vi "automatic_step_first_name.vi"(7 "transition_queue":refnum<queue>, 8 "error in (no error)":errorcluster, 10 "data":variant, 11 "recipe_data":variant) -> (0 "error out":errorcluster)   [LabVIEW 2015, in "example_02.lvlib"]
uses:
  example_02.lvlib
  <userlib>/antonio-alexander/lv-recipe-machine/public/_controls/transition.ctl
  _controls/customer.ctl
  <userlib>/antonio-alexander/lv-recipe-machine/lv-recipe-machine.lvlib
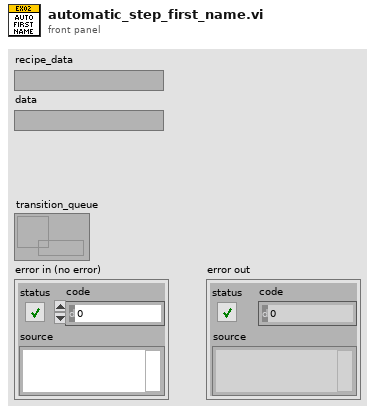
[diagram p1: front panel]
types:
  T1 = typedef "example_02.lvlib/customer.ctl" = cluster{"first_name":string, "last_name":string, "address_1":string, "address_2":string, "city":string, "state":string, "zip_code":string}
  T2 = typedef "example_02.lvlib/data.ctl" = cluster{"type":T3, "data":variant}
  T3 = typedef "example_02.lvlib/data_type.ctl" = enum16{"<data_type>", "first_name", "last_name", "address"}
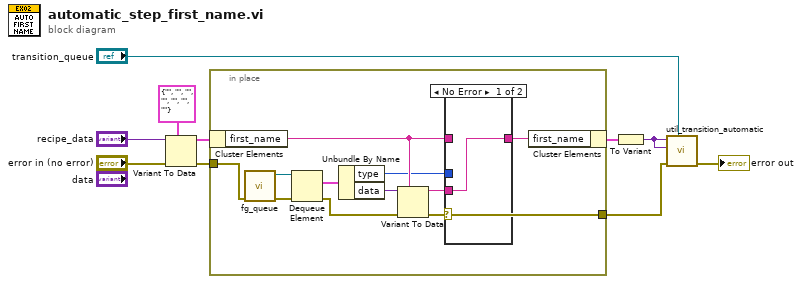
[diagram p0: block diagram]
diagram:
  n1 = Variant To Data(error in="error in (no error)", type=T1 {"first_name"="", "last_name"="", "address_1"="", "address_2"="", "city"="", "state"="", "zip_code"=""} ("customer"), Variant="recipe_data") -> (data=w5:T1, error out=w2:errorcluster)
  n2 = in-place {
    in-place-border: w2 -> [w19]
    in-place-border: [w14] -> w1
    n3 = in-place-cluster #1(w5) -> ("first_name"=w15:string)
    n4 = call "fg_queue.vi"("error in (no error)"=w19) -> ("error out"=w20:errorcluster, "queue out"=w21:refnum<queue>)  [unwired: 9 in]
    n5 = Dequeue Element(queue=w21, error in (no error)=w20) -> (element=w18:T2, error out=w16:errorcluster)  [unwired: 1 in, 2 out]
    n6 = Unbundle By Name(w18) -> ("type"=w11:T3, "data"=w17:variant)
    n7 = Variant To Data(error in=w16, type=w15, Variant=w17) -> (data=w13:string, error out=w14:errorcluster)
    n8 = case shown="No Error" w14 {
      tunnel: w15 -> [_ w23]
      tunnel: w13 -> [w22 _]
      tunnel: [w22 w23] -> w12
      tunnel: w11 -> [_ _]
      frame No Error {
      }
      frame Error {
      }
    }
    n9 = in-place-cluster #1("first_name"=w12) -> (w4:T1)
  }
  n10 = To Variant(anything=w4) -> (Variant=w3:variant)
  n11 = call <userlib>:"util_transition_automatic.vi"("transition_queue"="transition_queue", "error in (no error)"=w1, "data"=w3, "recipe_data"=w3) -> ("error out"=→"error out":errorcluster)  [unwired: 7 in]
